vi "Right Select Beacon Loop (SubVI).vi"   [LabVIEW 2015]
uses:
  Right Variables.vi
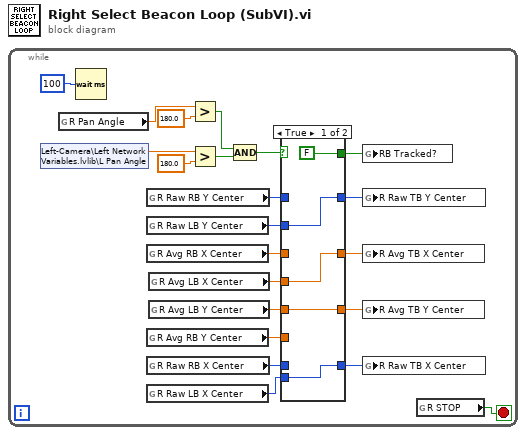
[diagram p0: block diagram]
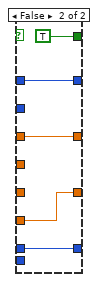
[diagram p2: hidden frame]
diagram:
  n1 = while {
    stop <- w15 stop-if-true
    n2 = shared-variable "Left-Camera\\Left Network Variables.lvlib\\L Pan Angle"() -> (w19:dbl)  [unwired: 1 in, 1 out]
    n3 = global read "Right Variables.vi" "R Pan Angle"() -> (w14:dbl)
    n4 = Wait (ms)(milliseconds to wait=u32 100) -> ()  [unwired: 1 out]
    n5 = global read "Right Variables.vi" "R Raw RB Y Center"() -> (w12:u16)
    n6 = global read "Right Variables.vi" "R Raw LB Y Center"() -> (w11:u16)
    n7 = global read "Right Variables.vi" "R Avg RB X Center"() -> (w10:dbl)
    n8 = global read "Right Variables.vi" "R Avg RB Y Center"() -> (w7:dbl)
    n9 = global read "Right Variables.vi" "R Raw RB X Center"() -> (w6:u16)
    n10 = global read "Right Variables.vi" "R Raw LB X Center"() -> (w5:u16)
    n11 = global read "Right Variables.vi" "R Avg LB X Center"() -> (w9:dbl)
    n12 = global read "Right Variables.vi" "R Avg LB Y Center"() -> (w8:dbl)
    n13 = Greater?(x=w14, y=180.0 ("upper limit")) -> (0:w21:bool)
    n14 = Greater?(x=w19, y=180.0 ("upper limit")) -> (0:w20:bool)
    n15 = Compound Arithmetic op=AND(w21, w20) -> (w22:bool)
    n16 = case shown="True" w22 {
      tunnel: [w27 w32] -> w4
      tunnel: w6 -> [_ w32]
      tunnel: w5 -> [w27 _]
      tunnel: [w26 w31] -> w2
      tunnel: w9 -> [w26 _]
      tunnel: w10 -> [_ w31]
      tunnel: [w25 w30] -> w3
      tunnel: w8 -> [w25 _]
      tunnel: w7 -> [_ w30]
      tunnel: [w24 w29] -> w1
      tunnel: w12 -> [_ w29]
      tunnel: w11 -> [w24 _]
      tunnel: [FALSE TRUE] -> w13
      frame True {
      }
      frame False {
      }
    }
    n17 = global write "Right Variables.vi" "RB Tracked?"(w13) -> ()
    n18 = global write "Right Variables.vi" "R Raw TB Y Center"(w1) -> ()
    n19 = global write "Right Variables.vi" "R Avg TB X Center"(w2) -> ()
    n20 = global write "Right Variables.vi" "R Avg TB Y Center"(w3) -> ()
    n21 = global write "Right Variables.vi" "R Raw TB X Center"(w4) -> ()
    n22 = global read "Right Variables.vi" "R STOP"() -> (w15:bool)
  }
